vi "Test Customer Update Order Number Broadcasts Order Number.vi"(8 "error in (no error)":errorcluster, 11 "Customer Test in":refnum<class "Customer Test.lvclass">) -> (0 "error out":errorcluster, 3 "Customer Test out":refnum<class "Customer Test.lvclass">)   [LabVIEW 2020, in "Customer Test.lvclass"]
uses:
  Customer Test.lvclass
  C:/Program Files (x86)/National Instruments/LabVIEW 2020/vi.lib/Astemes/LUnit/Test Case.lvclass
  Processes/People/Customers/Customer/Customer.lvclass
  C:/Program Files (x86)/National Instruments/LabVIEW 2020/vi.lib/Astemes/Triarc Framework/Process/Process.lvclass
  Processes/People/Customers/Customer/Public/Order State.ctl
  <vilib>/Astemes/Triarc Framework/Process/Process.lvclass/Process.ctl
  <vilib>/Astemes/LUnit/Test Case.lvclass/Test Case.ctl
  1c31fc30-13eb-4fa9-8415-74854b0cb702.vi
  <vilib>/Astemes/Triarc Framework/Process/Public/Lifecycle/Get Lifecycle State.vi
  <vilib>/Astemes/Triarc Framework/Broadcast Event Helpers/Execution timer.vi
  <vilib>/Astemes/Triarc Framework/Process/Private/SubVIs/Wait for finish.vi
  <vilib>/Astemes/Triarc Framework/Process/Private/SubVIs/Set Lifecycle State.vi
  <vilib>/Astemes/Triarc Framework/Process/Protected/Messaging/Send Message.vi
  <vilib>/Astemes/LUnit/Palette/Pass.vi
  <vilib>/Astemes/LUnit/Palette/Fail.vi
  <vilib>/Astemes/LUnit/Compare Variants.vi
  <vilib>/Astemes/LUnit/Describe Comparison.vi
  <vilib>/Astemes/LUnit/Set Assertion Type.vi
  <vilib>/Utility/error.llb/Clear Errors.vi
  <vilib>/Astemes/Triarc Framework/Process/Private/SubVIs/Handle Debug Data.vi
  <vilib>/Astemes/LUnit/Add test result.vi
  <vilib>/Astemes/LUnit/Variant to string.vi
  <vilib>/Astemes/Triarc Framework/Logging/Log Debug.vi
  <vilib>/AdvancedString/1D String Array to Delimited String.vi
  <vilib>/Utility/High Resolution Relative Seconds.vi
  <vilib>/Astemes/LUnit/LUnit Record Assertion Result.vi
  <vilib>/Astemes/LUnit/LUnit Aggregate Assertion Results.vi
  <vilib>/Astemes/LUnit/Method Result/LUnit Merge Status.vi
  <vilib>/Astemes/LUnit/LUnit Concatenate result strings.vi
  <vilib>/Utility/error.llb/Error Cluster From Error Code.vi
  <vilib>/Astemes/Triarc Framework/Broadcast Event Helpers/Dequeue Broadcast Message.vi
  <vilib>/Astemes/Triarc Framework/Process/Public/Read Name.vi
  <vilib>/Utility/Data Type/Get Type Information.vi
  <vilib>/Utility/LVClass/Get LV Class Name.vi
  <vilib>/Astemes/Triarc Framework/Process/Process.lvclass
  <vilib>/Astemes/Triarc Framework/Broadcast Event Helpers/Broadcast Event Helpers.lvlib
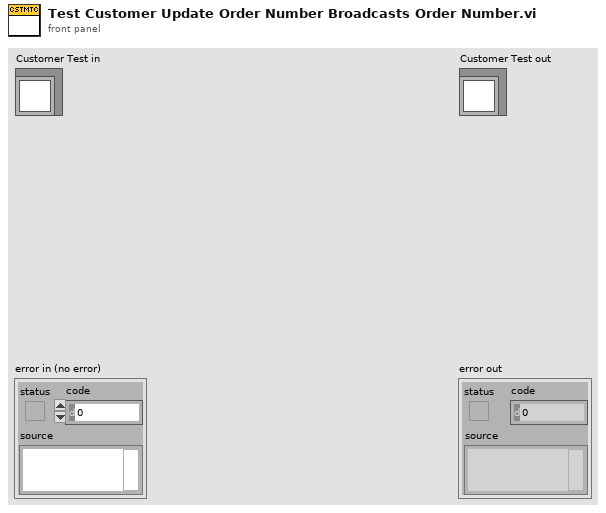
[diagram p1: front panel]
types:
  T1 = typedef "Customer.lvclass/Order State.ctl" = cluster{"Order In Progress?":bool, "Order Number":u32, "Order Price":dbl, "Items Ordered":u32, "Items Received":u32, "Items Picked Up":string}
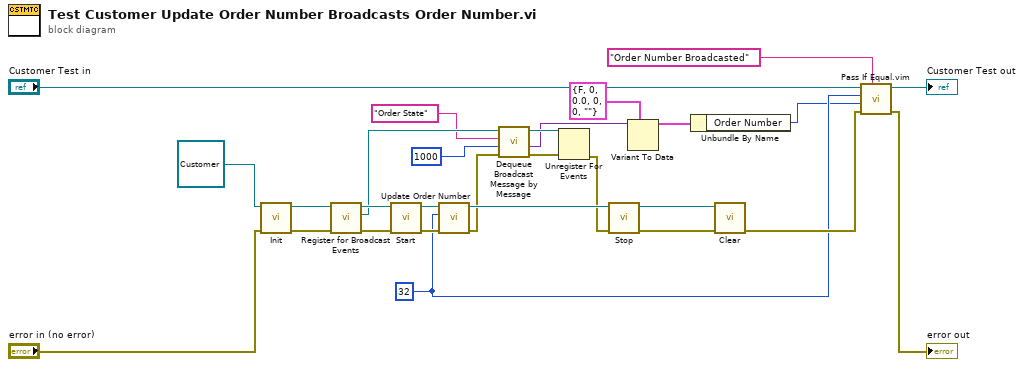
[diagram p0: block diagram]
diagram:
  w5 = u32 32 ("Order Number")
  n1 = call-dynamic "Init.vi"("error in (no error)"="error in (no error)", "View In"=refnum<class "Customer.lvclass"> refnum ("Customer.lvclass")) -> ("error out"=w24:errorcluster, "View Out"=w25:refnum<class "Customer.lvclass">)  [unwired: 8 in]
  n2 = call <vilib>:"Register for Broadcast Events.vi"("error in (no error)"=w24, "Process In"=w25) -> ("error out"=w27:errorcluster, "Event Registration Refnum Out"=w20:refnum<event-registration>, "Process Out"=w26:refnum<class "Customer.lvclass">)  [unwired: 7 in]
  n3 = call <vilib>:"Start.vi"("error in (no error)"=w27, "Process In"=w26) -> ("error out"=w17:errorcluster, "Process Out"=w19:refnum<class "Customer.lvclass">)  [unwired: 7 in, 1 out]
  n4 = call "Update Order Number.vi"("error in (no error)"=w17, "Order Number"=w5, "Customer In"=w19) -> ("error out"=w16:errorcluster, "Customer Out"=w18:refnum<class "Customer.lvclass">)  [unwired: 7 in]
  n5 = call <vilib>:"Dequeue Broadcast Message by Message.vi"("error in (no error)"=w16, "Timeout (-1)"=1000, "Message"="Order State", "Event Registration Refnum"=w20) -> ("error out"=w15:errorcluster, "Message Data"=w2:variant, "Event Registration Refnum Out"=w8:refnum<event-registration>)  [unwired: 3 in, 2 out]
  n6 = Unregister For Events(event registration refnum=w8, error in=w15) -> (error out=w12:errorcluster)
  n7 = call <vilib>:"Stop.vi"("error in (no error)"=w12, "Process In"=w18) -> ("error out"=w22:errorcluster, "Process Out"=w23:refnum<class "Customer.lvclass">)  [unwired: 7 in, 1 out]
  n8 = Variant To Data(type=T1 {"Order In Progress?"=FALSE, "Order Number"=0, "Order Price"=0.0, "Items Ordered"=0, "Items Received"=0, "Items Picked Up"=""} ("Order State"), Variant=w2) -> (data=w3:T1)  [unwired: 1 in, 1 out]
  n9 = Unbundle By Name(w3) -> ("Order Number"=w1:u32)
  n10 = call-dynamic "Clear.vi"("error in (no error)"=w22, "View In"=w23) -> ("error out"=w11:errorcluster)  [unwired: 9 in]
  n11 = call "Pass If Equal.vim"("Description"="Order Number Broadcasted", "error in (no error)"=w11, "Actual"=w1, "Expected"=w5, "LUnit Test Case In"="Customer Test in") -> ("error out"=→"error out":errorcluster, "LUnit Test Case Out"=→"Customer Test out":refnum<class "Customer Test.lvclass">)  [unwired: 5 in]
